vi "SubPanel - Symmetrical Components Analysis.vi"() -> ()   [LabVIEW 2021]
uses:
  <vilib>/Analysis/5stat.llb/RMS (DBL).vi
  <vilib>/measure/matone.llb/Extract Single Tone Information 1 Chan.vi
  <vilib>/Analysis/NI_AALPro.lvlib
  <vilib>/measure/NI_MAPro.lvlib
panel:
  out "I0 L1 Phase":cdb=-0.5+0.8860254i format="%#_13g"
  out "I0 L2 Phase":cdb=-0.5+0.8860254i format="%#_13g"
  out "I0 L3 Phase":cdb=-0.5+0.8860254i format="%#_13g"
  out "I+ L1 Phase":cdb=-0.5+0.8860254i format="%#_13g"
  out "I+ L2 Phase":cdb=-0.5+0.8860254i format="%#_13g"
  out "I+ L3 Phase":cdb=-0.5+0.8860254i format="%#_13g"
  out "I- L1 Phase":cdb=-0.5+0.8860254i format="%#_13g"
  out "I- L2 Phase":cdb=-0.5+0.8860254i format="%#_13g"
  out "I- L3 Phase":cdb=-0.5+0.8860254i format="%#_13g"
  out "V- L1 Phase":cdb=-0.5+0.8860254i format="%#_13g"
  out "V- L2 Phase":cdb=-0.5+0.8860254i format="%#_13g"
  out "V- L3 Phase":cdb=-0.5+0.8860254i format="%#_13g"
  out "V+ L1 Phase":cdb=-0.5+0.8860254i format="%#_13g"
  out "V+ L2 Phase":cdb=-0.5+0.8860254i format="%#_13g"
  out "V+ L3 Phase":cdb=-0.5+0.8860254i format="%#_13g"
  out "V0 L3 Phase":cdb=-0.5+0.8860254i format="%#_13g"
  out "V0 L2 Phase":cdb=-0.5+0.8860254i format="%#_13g"
  out "V0 L1 Phase":cdb=-0.5+0.8860254i format="%#_13g"
  out "error out":errorcluster
  in  "error in":errorcluster
  in  "Samples per Channel":i32
  out "Currents":dbl[][](graph)
  out "Phases Shifts":T1
  out "Phase L3":T2 {"U-I Phase Shift" format="%#.3f"}
  out "Phase L2":T2 {"U-I Phase Shift" format="%#.3f"}
  out "Phase L1":T2 {"U-I Phase Shift" format="%#.3f"; "Initial Current Angle" format="%#.3f"; "Initial Voltage Angle" format="%#.3f"}
  out "Voltages":dbl[][](graph)
  # "L1"
  # "L2"
  # "L3"
  # "deg"
  # "deg"
  # "deg"
  # "deg"
  # "deg"
  # "deg"
  # "V"
  # "A"
  # "deg"
  # "deg"
  # "deg"
  # "A"
  # "deg"
  # "deg"
  # "deg"
  # "V"
  # "A"
  # "deg"
  # "deg"
  # "deg"
  # "V"
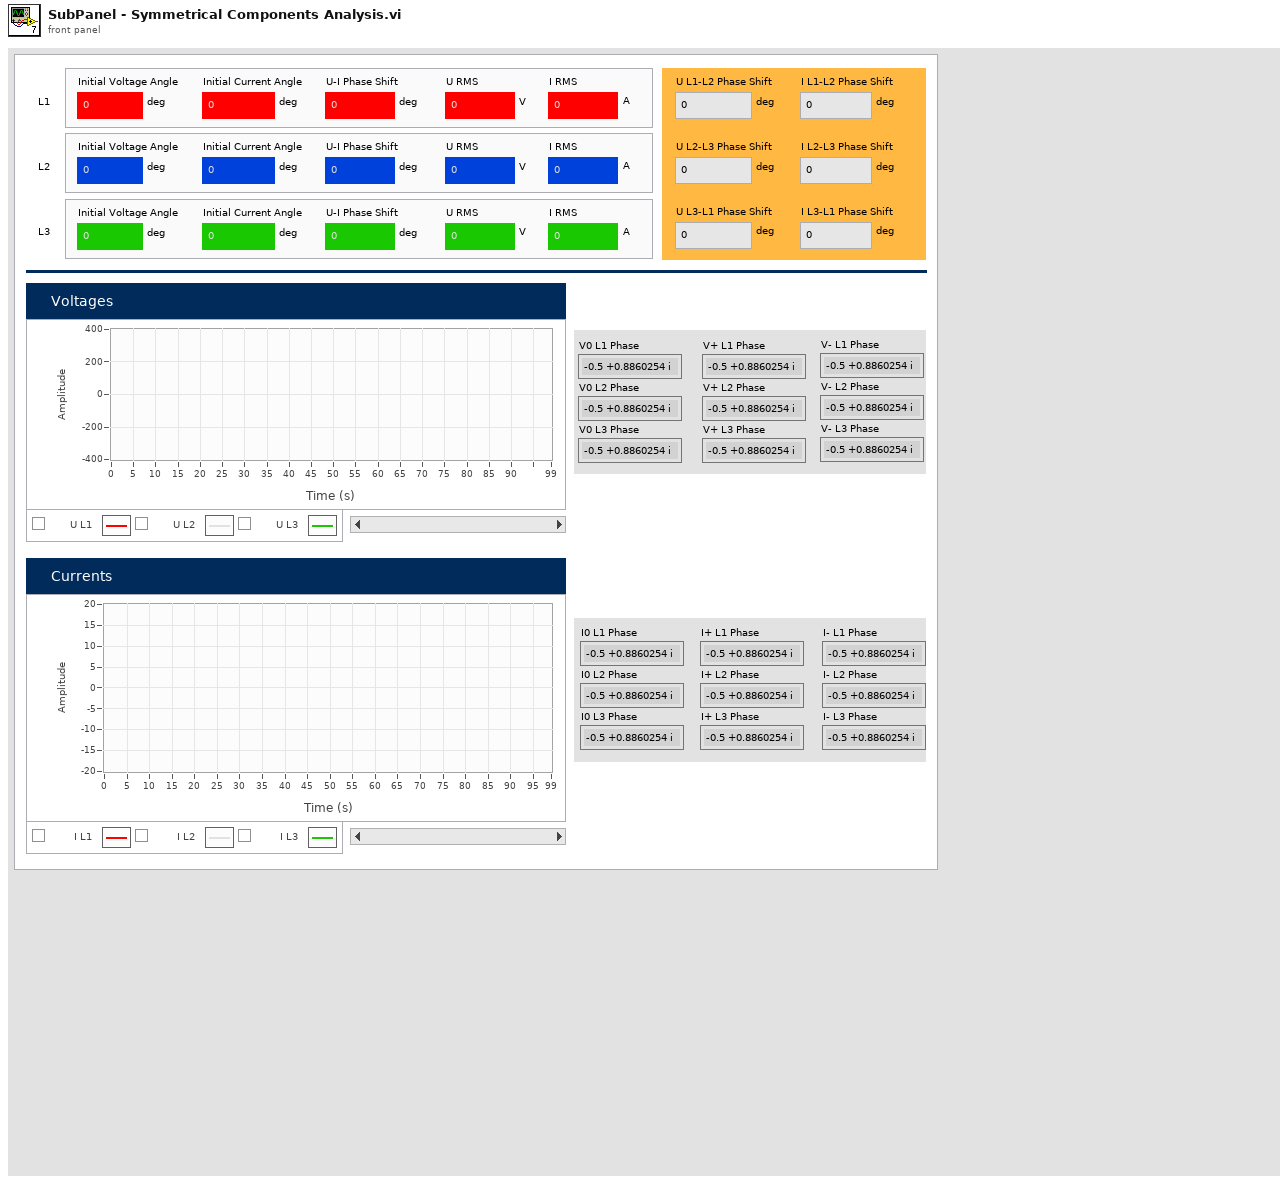
[diagram p1: front panel]
types:
  T1 = cluster{"U L1-L2 Phase Shift":dbl, "U L2-L3 Phase Shift":dbl, "U L3-L1 Phase Shift":dbl, "I L1-L2 Phase Shift":dbl, "I L2-L3 Phase Shift":dbl, "I L3-L1 Phase Shift":dbl}
  T2 = cluster{"Initial Voltage Angle":dbl, "Initial Current Angle":dbl, "U-I Phase Shift":dbl, "U RMS":dbl, "I RMS":dbl}
  T3 = typedef "Message FPGA.ctl" = cluster{"Channel 1 Data (L1 U)":dbl[], "Channel 2 Data (L1 I)":dbl[], "Channel 3 Data (L2 U)":dbl[], "Channel 4 Data (L2 I)":dbl[], "Channel 5 Data (L3 U)":dbl[], "Channel 6 Data (L3 I)":dbl[]}
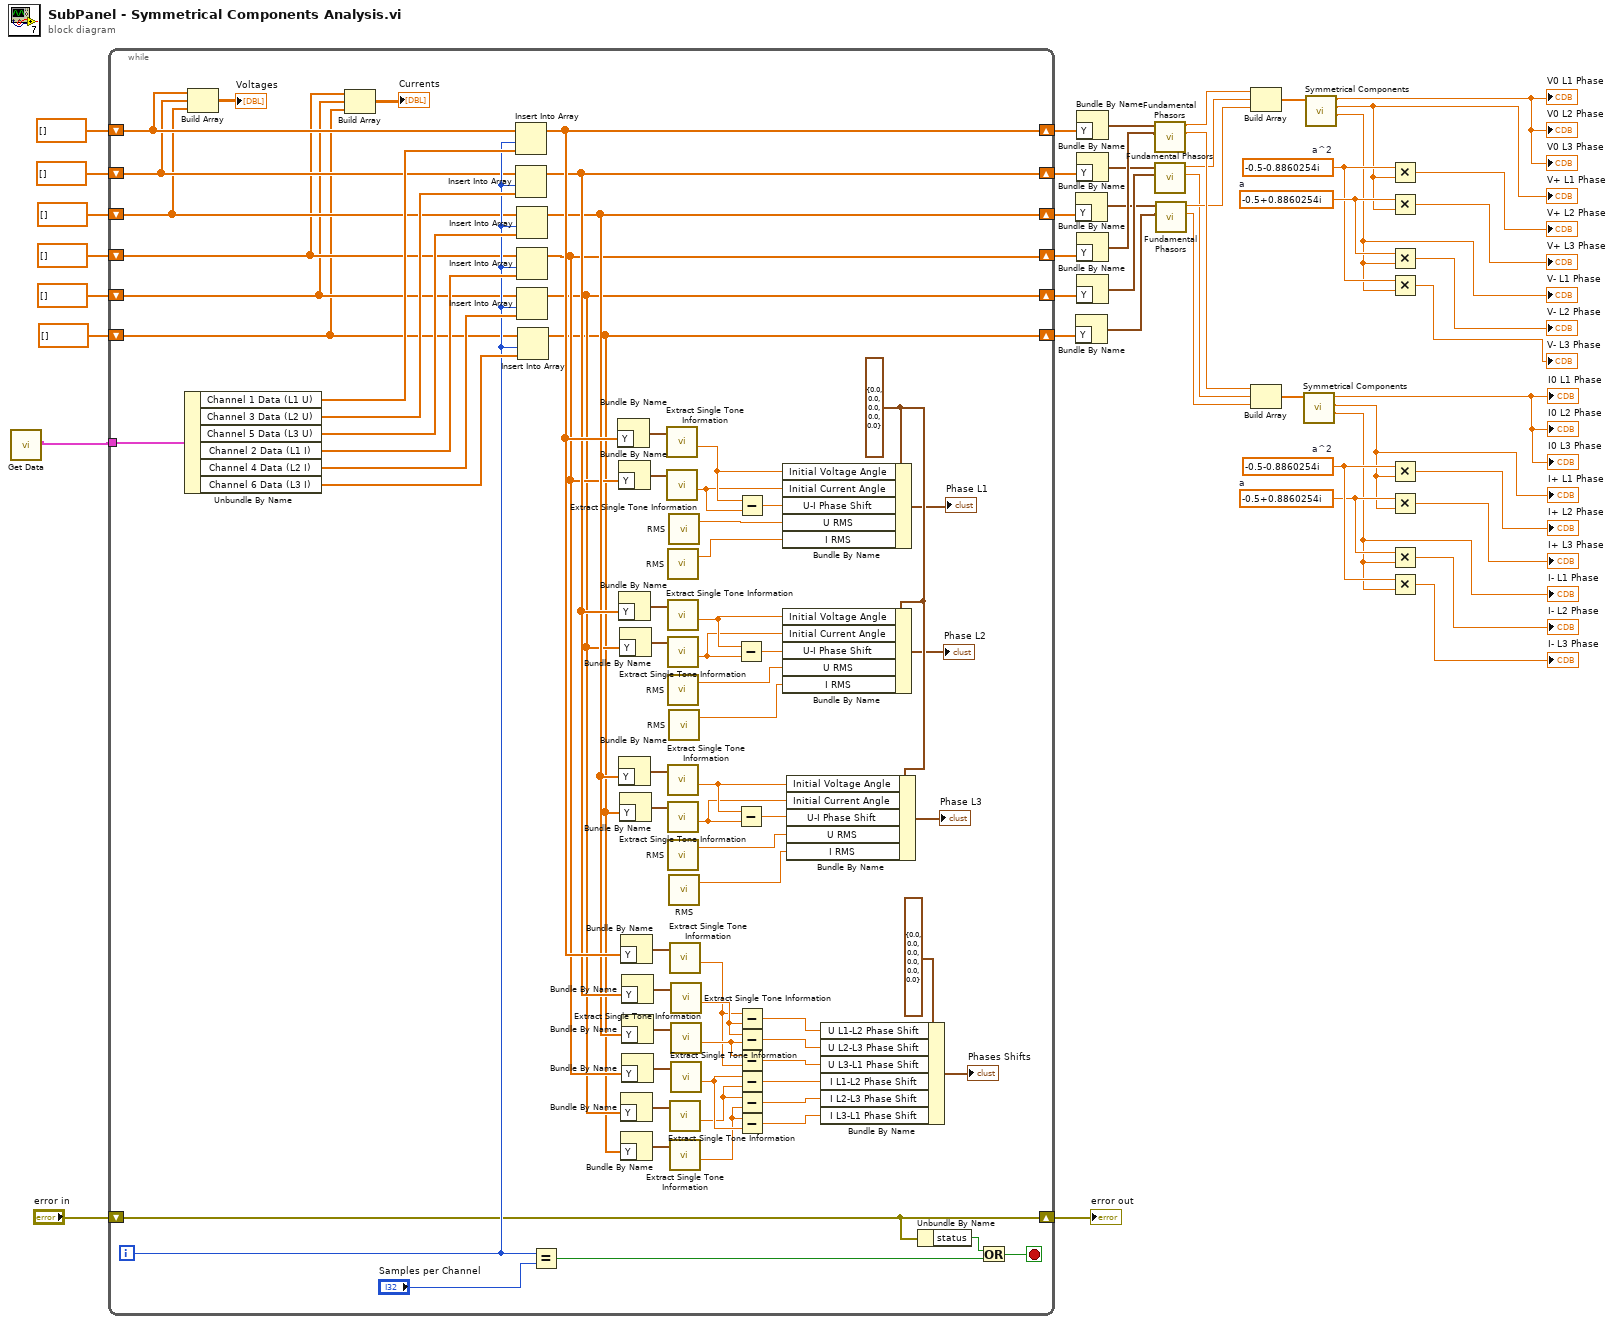
[diagram p0: block diagram]
diagram:
  w37 = cdb -0.5-0.8860254i  # a^2
  w36 = cdb -0.5+0.8860254i  # a
  w38 = cdb -0.5-0.8860254i  # a^2
  w39 = cdb -0.5+0.8860254i  # a
  n1 = call "Get Data.vi"() -> ("Message FPGA"=w1:T3)  [unwired: 10 in, 1 out]
  n2 = while {
    tunnel: w1 -> [w119]
    shift-right: [w54] -> w35
    shift-left: dbl[] [] -> [w107]
    shift-right: [w53] -> w34
    shift-left: dbl[] [] -> [w106]
    shift-right: [w52] -> w33
    shift-left: dbl[] [] -> [w105]
    shift-right: [w51] -> w32
    shift-left: dbl[] [] -> [w104]
    shift-right: [w50] -> w31
    shift-left: dbl[] [] -> [w103]
    shift-right: [w49] -> w30
    shift-left: dbl[] [] -> [w102]
    shift-right: [w58] -> w40
    shift-left: "error in" -> [w58]
    i -> [w112]
    stop <- w110 stop-if-true
    w99 = T2 {"Initial Voltage Angle"=0.0, "Initial Current Angle"=0.0, "U-I Phase Shift"=0.0, "U RMS"=0.0, "I RMS"=0.0} ("Phase L1")
    n3 = Unbundle By Name(w119) -> ("Channel 1 Data (L1 U)"=w118:dbl[], "Channel 3 Data (L2 U)"=w117:dbl[], "Channel 5 Data (L3 U)"=w116:dbl[], "Channel 2 Data (L1 I)"=w115:dbl[], "Channel 4 Data (L2 I)"=w114:dbl[], "Channel 6 Data (L3 I)"=w113:dbl[])
    n4 = Build Array(w107, w106, w105) -> (→"Voltages":dbl[][])
    n5 = Build Array(w104, w103, w102) -> (→"Currents":dbl[][])
    n6 = Insert Into Array(array=w107, index=w112, new element=w118) -> (w54:dbl[])
    n7 = Insert Into Array(array=w106, index=w112, new element=w117) -> (w53:dbl[])
    n8 = Insert Into Array(array=w105, index=w112, new element=w116) -> (w52:dbl[])
    n9 = Insert Into Array(array=w104, index=w112, new element=w115) -> (w51:dbl[])
    n10 = Insert Into Array(array=w103, index=w112, new element=w114) -> (w50:dbl[])
    n11 = Insert Into Array(array=w102, index=w112, new element=w113) -> (w49:dbl[])
    n12 = Equal?(x=w112, y="Samples per Channel") -> (x = y?=w108:bool)
    n13 = Bundle By Name("Y"=w54) -> (w96:waveform(dbl))  [unwired: 1 in]
    n14 = Bundle By Name("Y"=w51) -> (w95:waveform(dbl))  [unwired: 1 in]
    n15 = Bundle By Name("Y"=w53) -> (w74:waveform(dbl))  [unwired: 1 in]
    n16 = Bundle By Name("Y"=w52) -> (w68:waveform(dbl))  [unwired: 1 in]
    n17 = Bundle By Name("Y"=w50) -> (w75:waveform(dbl))  [unwired: 1 in]
    n18 = Bundle By Name("Y"=w49) -> (w67:waveform(dbl))  [unwired: 1 in]
    n19 = Bundle By Name("Y"=w54) -> (w86:waveform(dbl))  [unwired: 1 in]
    n20 = Bundle By Name("Y"=w50) -> (w89:waveform(dbl))  [unwired: 1 in]
    n21 = Bundle By Name("Y"=w49) -> (w88:waveform(dbl))  [unwired: 1 in]
    n22 = Bundle By Name("Y"=w53) -> (w87:waveform(dbl))  [unwired: 1 in]
    n23 = Bundle By Name("Y"=w52) -> (w91:waveform(dbl))  [unwired: 1 in]
    n24 = Bundle By Name("Y"=w51) -> (w90:waveform(dbl))  [unwired: 1 in]
    n25 = call-poly <vilib>:"Extract Single Tone Information.vi"("time signal in"=w96) -> ("detected phase (deg)"=w94:dbl)  [unwired: 5 in, 5 out]
    n26 = call-poly <vilib>:"Extract Single Tone Information.vi"("time signal in"=w95) -> ("detected phase (deg)"=w93:dbl)  [unwired: 5 in, 5 out]
    n27 = call-poly <vilib>:"RMS.vi"() -> ("rms value"=w97:dbl)  [unwired: 1 in, 1 out]
    n28 = call-poly <vilib>:"Extract Single Tone Information.vi"("time signal in"=w74) -> ("detected phase (deg)"=w73:dbl)  [unwired: 5 in, 5 out]
    n29 = call-poly <vilib>:"Extract Single Tone Information.vi"("time signal in"=w75) -> ("detected phase (deg)"=w72:dbl)  [unwired: 5 in, 5 out]
    n30 = call-poly <vilib>:"RMS.vi"() -> ("rms value"=w70:dbl)  [unwired: 1 in, 1 out]
    n31 = call-poly <vilib>:"Extract Single Tone Information.vi"("time signal in"=w68) -> ("detected phase (deg)"=w60:dbl)  [unwired: 5 in, 5 out]
    n32 = call-poly <vilib>:"Extract Single Tone Information.vi"("time signal in"=w67) -> ("detected phase (deg)"=w59:dbl)  [unwired: 5 in, 5 out]
    n33 = call-poly <vilib>:"RMS.vi"() -> ("rms value"=w65:dbl)  [unwired: 1 in, 1 out]
    n34 = call-poly <vilib>:"RMS.vi"() -> ("rms value"=w98:dbl)  [unwired: 1 in, 1 out]
    n35 = call-poly <vilib>:"RMS.vi"() -> ("rms value"=w69:dbl)  [unwired: 1 in, 1 out]
    n36 = call-poly <vilib>:"RMS.vi"() -> ("rms value"=w64:dbl)  [unwired: 1 in, 1 out]
    n37 = call-poly <vilib>:"Extract Single Tone Information.vi"("time signal in"=w86) -> ("detected phase (deg)"=w61:dbl)  [unwired: 5 in, 5 out]
    n38 = call-poly <vilib>:"Extract Single Tone Information.vi"("time signal in"=w89) -> ("detected phase (deg)"=w77:dbl)  [unwired: 5 in, 5 out]
    n39 = call-poly <vilib>:"Extract Single Tone Information.vi"("time signal in"=w88) -> ("detected phase (deg)"=w76:dbl)  [unwired: 5 in, 5 out]
    n40 = call-poly <vilib>:"Extract Single Tone Information.vi"("time signal in"=w87) -> ("detected phase (deg)"=w79:dbl)  [unwired: 5 in, 5 out]
    n41 = call-poly <vilib>:"Extract Single Tone Information.vi"("time signal in"=w91) -> ("detected phase (deg)"=w62:dbl)  [unwired: 5 in, 5 out]
    n42 = call-poly <vilib>:"Extract Single Tone Information.vi"("time signal in"=w90) -> ("detected phase (deg)"=w78:dbl)  [unwired: 5 in, 5 out]
    n43 = Subtract(x=w73, y=w72) -> (x-y=w71:dbl)
    n44 = Subtract(x=w60, y=w59) -> (x-y=w66:dbl)
    n45 = Subtract(x=w94, y=w93) -> (x-y=w63:dbl)
    n46 = Subtract(x=w61, y=w79) -> (x-y=w82:dbl)
    n47 = Subtract(x=w79, y=w62) -> (x-y=w83:dbl)
    n48 = Subtract(x=w62, y=w61) -> (x-y=w85:dbl)
    n49 = Subtract(x=w78, y=w77) -> (x-y=w84:dbl)
    n50 = Subtract(x=w77, y=w76) -> (x-y=w81:dbl)
    n51 = Subtract(x=w76, y=w78) -> (x-y=w80:dbl)
    n52 = Bundle By Name(cluster=w99, "Initial Voltage Angle"=w94, "Initial Current Angle"=w93, "U-I Phase Shift"=w63, "U RMS"=w98, "I RMS"=w97) -> (→"Phase L1":T2)
    n53 = Bundle By Name(cluster=w99, "Initial Voltage Angle"=w73, "Initial Current Angle"=w72, "U-I Phase Shift"=w71, "U RMS"=w70, "I RMS"=w69) -> (→"Phase L2":T2)
    n54 = Bundle By Name(cluster=w99, "Initial Voltage Angle"=w60, "Initial Current Angle"=w59, "U-I Phase Shift"=w66, "U RMS"=w65, "I RMS"=w64) -> (→"Phase L3":T2)
    n55 = Bundle By Name(cluster=T1 {"U L1-L2 Phase Shift"=0.0, "U L2-L3 Phase Shift"=0.0, "U L3-L1 Phase Shift"=0.0, "I L1-L2 Phase Shift"=0.0, "I L2-L3 Phase Shift"=0.0, "I L3-L1 Phase Shift"=0.0} ("Phases Shifts"), "U L1-L2 Phase Shift"=w82, "U L2-L3 Phase Shift"=w83, "U L3-L1 Phase Shift"=w85, "I L1-L2 Phase Shift"=w84, "I L2-L3 Phase Shift"=w81, "I L3-L1 Phase Shift"=w80) -> (→"Phases Shifts":T1)
    n56 = Unbundle By Name(w58) -> ("status"=w109:bool)
    n57 = Or(x=w109, y=w108) -> (x .or. y?=w110:bool)
  }
  "error out" <- w40
  n58 = Bundle By Name("Y"=w33) -> (w23:waveform(dbl))  [unwired: 1 in]
  n59 = Bundle By Name("Y"=w30) -> (w22:waveform(dbl))  [unwired: 1 in]
  n60 = Bundle By Name("Y"=w35) -> (w29:waveform(dbl))  [unwired: 1 in]
  n61 = Bundle By Name("Y"=w34) -> (w25:waveform(dbl))  [unwired: 1 in]
  n62 = Bundle By Name("Y"=w32) -> (w28:waveform(dbl))  [unwired: 1 in]
  n63 = Bundle By Name("Y"=w31) -> (w24:waveform(dbl))  [unwired: 1 in]
  n64 = call "Fundamental Phasors.vi"("current waveform"=w28, "voltage waveform"=w29) -> ("current fundamental vector"=w26:cdb, "voltage fundamental vector"=w27:cdb)  [unwired: 6 in, 2 out]
  n65 = call "Fundamental Phasors.vi"("current waveform"=w24, "voltage waveform"=w25) -> ("current fundamental vector"=w17:cdb, "voltage fundamental vector"=w19:cdb)  [unwired: 6 in, 2 out]
  n66 = call "Fundamental Phasors.vi"("current waveform"=w22, "voltage waveform"=w23) -> ("current fundamental vector"=w16:cdb, "voltage fundamental vector"=w18:cdb)  [unwired: 6 in, 2 out]
  n67 = Build Array(w27, w19, w18) -> (w21:cdb[])
  n68 = Build Array(w26, w17, w16) -> (w20:cdb[])
  n69 = call "Symmetrical Components.vi"("3-phase phasors"=w20) -> ("zero sequence"=w4:cdb, "negative sequence"=w7:cdb, "positive sequence"=→"I0 L1 Phase" →"I0 L2 Phase" →"I0 L3 Phase":cdb)  [unwired: 7 in, 1 out]
  "I+ L1 Phase" <- w7
  "I- L1 Phase" <- w4
  n70 = call "Symmetrical Components.vi"("3-phase phasors"=w21) -> ("zero sequence"=w11:cdb, "negative sequence"=w14:cdb, "positive sequence"=→"V0 L1 Phase" →"V0 L2 Phase" →"V0 L3 Phase":cdb)  [unwired: 7 in, 1 out]
  "V+ L1 Phase" <- w14
  "V- L1 Phase" <- w11
  n71 = Multiply(x=w38, y=w14) -> (x*y=→"V+ L2 Phase":cdb)
  n72 = Multiply(x=w39, y=w14) -> (x*y=→"V+ L3 Phase":cdb)
  n73 = Multiply(x=w39, y=w11) -> (x*y=→"V- L2 Phase":cdb)
  n74 = Multiply(x=w38, y=w11) -> (x*y=→"V- L3 Phase":cdb)
  n75 = Multiply(x=w37, y=w7) -> (x*y=→"I+ L2 Phase":cdb)
  n76 = Multiply(x=w36, y=w7) -> (x*y=→"I+ L3 Phase":cdb)
  n77 = Multiply(x=w36, y=w4) -> (x*y=→"I- L2 Phase":cdb)
  n78 = Multiply(x=w37, y=w4) -> (x*y=→"I- L3 Phase":cdb)
